vi "Swerve Drive 6181.vi"(0 "X":dbl(slide) scale=-1.0..1.0, 1 "Y":dbl(slide) scale=1.0..-1.0, 2 "Z":dbl(knob) scale=1.0..-1.0, 3 "Robot-Centric":bool, 4 "Auto Controls":bool) -> (5 "Avg Sensor Pos":dbl)   [LabVIEW 2019]
panel:
  in  "Robot Length":dbl=21.5
  in  "Robot Width":dbl=29.5
  # "SWERVE DRIVE\nVersion 3.1\n\nCory Lynch\nApple Pi Robotics\nTeam 2067"
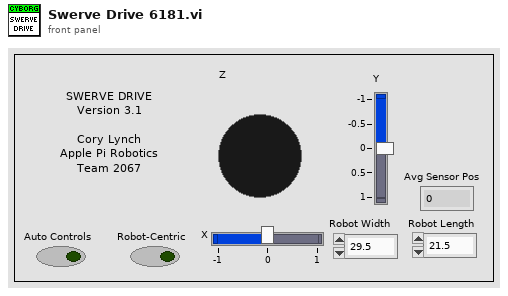
[diagram p1: front panel]
types:
  T1 = enum16{"Back Left", "Back Right", "Front Left", "Front Right"}
  T2 = cluster{"Yaw":dbl, "Roll":dbl, "Pitch":dbl, "Heading":dbl, "Fused Heading":dbl}
  T3 = typedef "WPI_MotorControlDeviceRef.ctl" = cluster{"DeviceStatus":errorcluster, "Type":T4, "PWM":cluster{"PWM Channel":T5, "DeadBand":T6}, "CAN":cluster{"Device Number":u8, "SetOutput VI Ref":variant, "GetOutput VI Ref":variant, "Enable VI Ref":variant, "Disable VI Ref":variant, "Data":variant}, "Invert":bool, "DIO PWM":cluster{"PWM \"Enable\" Channel":T5, "DIOChannel":T7, "PWM Rate":dbl}}
  T4 = typedef "WPI_MotorControlType.ctl" = enum16{"PWM", "CAN", "DIO PWM"}
  T5 = typedef "FPGA_DIOPWMChannel.ctl" = enum8{"PWM 0", "PWM 1", "PWM 2", "PWM 3", "PWM 4", "PWM 5", "PWM 6", "PWM 7", "PWM 8", "PWM 9", "PWM MXP 0", "PWM MXP 1", "PWM MXP 2", "PWM MXP 3", "PWM MXP 4", "PWM MXP 5", "PWM MXP 6", "PWM MXP 7", "PWM MXP 8", "PWM MXP 9", "Invalid"}
  T6 = typedef "WPI_PWMDeadband.ctl" = cluster{"Name":string, "maxPositivePwm":i32, "minPositivePwm":i32, "centerPwm":i32, "maxNegativePwm":i32, "minNegativePwm":i32, "angularRange":u16}
  T7 = typedef "FPGA_DIOChannel.ctl" = enum8{"DIO 0", "DIO 1", "DIO 2", "DIO 3", "DIO 4", "DIO 5", "DIO 6", "DIO 7", "DIO 8", "DIO 9", "DIO MXP 0", "DIO MXP 1", "DIO MXP 2", "DIO MXP 3", "DIO MXP 4", "DIO MXP 5", "DIO MXP 6", "DIO MXP 7", "DIO MXP 8", "DIO MXP 9", "DIO MXP 10", "DIO MXP 11", "DIO MXP 12", "DIO MXP 13", "DIO MXP 14", "DIO MXP 15", "SPI Port CS1", "SPI Port CS2", "SPI Port CS3", "SPI Port MISO", "SPI Port MOSI", "Invalid"}
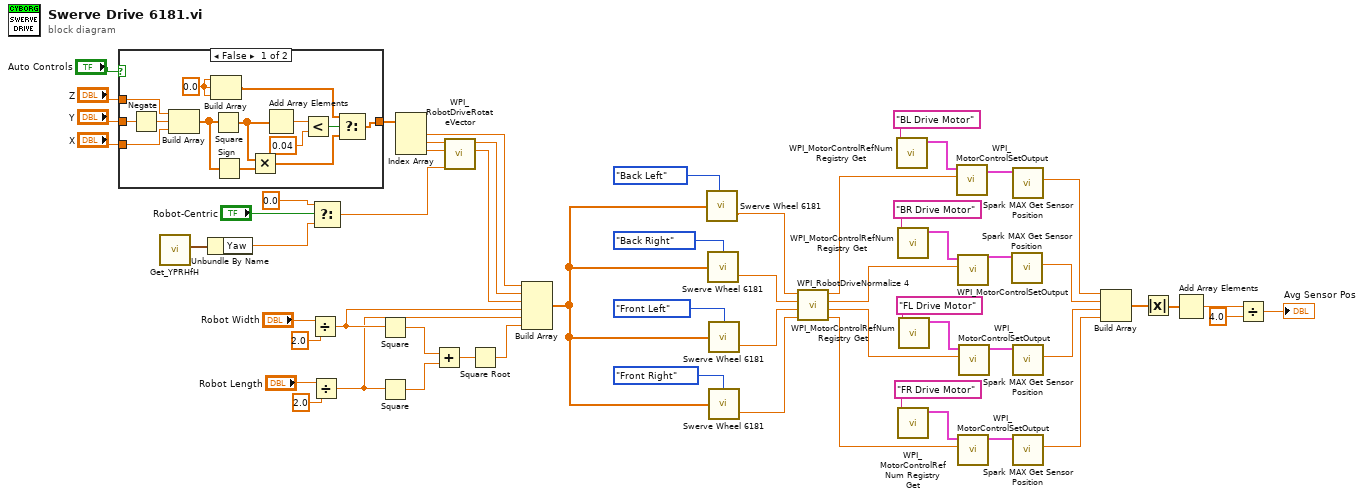
[diagram p0: block diagram]
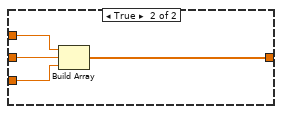
[diagram p2: hidden frame]
diagram:
  n1 = case shown="False" "Auto Controls" {
    tunnel: "Y" -> [w70 w76]
    tunnel: "X" -> [w64 w77]
    tunnel: "Z" -> [w60 w74]
    tunnel: [w61 w75] -> w35
    frame False {
      w68 = 0.0 ("element")
      n2 = Negate(x=w70) -> (-x=w63:dbl)
      n3 = Build Array(w60, w63, w64) -> (w67:dbl[])
      n4 = Build Array(w68, w68, w68) -> (w69:dbl[])
      n5 = Square(x=w67) -> (x^2=w65:dbl[])
      n6 = Sign(1:w67) -> (0:w66:dbl[])
      n7 = Multiply(x=w65, y=w66) -> (x*y=w62:dbl[])
      n8 = Add Array Elements(numeric array=w65) -> (sum=w73:dbl)
      n9 = Less?(x=w73, y=0.04 ("x")) -> (x < y?=w71:bool)
      n10 = Select(t=w69, s=w71, f=w62) -> (s? t:f=w61:dbl[])
    }
    frame True {
      n11 = Build Array(w74, w76, w77) -> (w75:dbl[])
    }
  }
  n12 = call <vilib>:"Get_YPRHfH.vi"() -> ("YRPHfH"=w26:T2)  [unwired: 11 in]
  n13 = Unbundle By Name(w26) -> ("Yaw"=w27:dbl)
  n14 = Divide(x="Robot Width", y=2.0) -> (x/y=w25:dbl)
  n15 = Divide(x="Robot Length", y=2.0) -> (x/y=w24:dbl)
  n16 = Select(t=0.0, s="Robot-Centric", f=w27) -> (s? t:f=w32:dbl)
  n17 = Square(x=w25) -> (x^2=w45:dbl)
  n18 = Square(x=w24) -> (x^2=w46:dbl)
  n19 = Index Array(array=w35) -> (element #1=w31:dbl, element #2=w36:dbl, element #3=w39:dbl)  [unwired: 3 in]
  n20 = Add(x=w45, y=w46) -> (x+y=w44:dbl)
  n21 = call <vilib>:"WPI_RobotDriveRotateVector.vi"("Angle"=w32, "X"=w39, "Y"=w36) -> ("X'"=w34:dbl, "Y'"=w30:dbl)  [unwired: 7 out]
  n22 = Square Root(x=w44) -> (sqrt(x)=w23:dbl)
  n23 = Build Array(w31, w30, w34, w25, w24, w23) -> (w15:dbl[])
  n24 = call "Swerve Wheel 6181.vi"("Wheel"=T1."Back Left", "Inputs"=w15) -> ("Speed"=w22:dbl)  [unwired: 3 in]
  n25 = call "Swerve Wheel 6181.vi"("Wheel"=T1."Back Right", "Inputs"=w15) -> ("Speed"=w20:dbl)  [unwired: 3 in]
  n26 = call "Swerve Wheel 6181.vi"("Wheel"=T1."Front Left", "Inputs"=w15) -> ("Speed"=w18:dbl)  [unwired: 3 in]
  n27 = call "Swerve Wheel 6181.vi"("Wheel"=T1."Front Right", "Inputs"=w15) -> ("Speed"=w16:dbl)  [unwired: 3 in]
  n28 = call <vilib>:"WPI_RobotDriveNormalize 4.vi"("D"=w16, "C"=w18, "B"=w20, "A"=w22) -> ("D'"=w48:dbl, "C'"=w49:dbl, "B'"=w50:dbl, "A'"=w51:dbl)
  n29 = call <vilib>:"WPI_MotorControlRefNum Registry Get.vi"("refnum name"="BL Drive Motor") -> ("MotorControlDevRef"=w59:T3)  [unwired: 9 in, 1 out]
  n30 = call <vilib>:"WPI_MotorControlRefNum Registry Get.vi"("refnum name"="BR Drive Motor") -> ("MotorControlDevRef"=w56:T3)  [unwired: 9 in, 1 out]
  n31 = call <vilib>:"WPI_MotorControlRefNum Registry Get.vi"("refnum name"="FR Drive Motor") -> ("MotorControlDevRef"=w52:T3)  [unwired: 9 in, 1 out]
  n32 = call <vilib>:"WPI_MotorControlRefNum Registry Get.vi"("refnum name"="FL Drive Motor") -> ("MotorControlDevRef"=w55:T3)  [unwired: 9 in, 1 out]
  n33 = call <vilib>:"WPI_MotorControlSetOutput.vi"("Output"=w51, "MotorControlDevRef"=w59) -> ("MotorControlDevRef"=w13:T3)  [unwired: 7 in, 2 out]
  n34 = call <vilib>:"WPI_MotorControlSetOutput.vi"("Output"=w50, "MotorControlDevRef"=w56) -> ("MotorControlDevRef"=w12:T3)  [unwired: 7 in, 2 out]
  n35 = call <vilib>:"WPI_MotorControlSetOutput.vi"("Output"=w48, "MotorControlDevRef"=w52) -> ("MotorControlDevRef"=w10:T3)  [unwired: 7 in, 2 out]
  n36 = call <vilib>:"WPI_MotorControlSetOutput.vi"("Output"=w49, "MotorControlDevRef"=w55) -> ("MotorControlDevRef"=w11:T3)  [unwired: 7 in, 2 out]
  n37 = call <vilib>:"Spark MAX Get Sensor Position.vi"("MotorControlDevRef in"=w12) -> ("Sensor Position"=w7:dbl)  [unwired: 7 in, 3 out]
  n38 = call <vilib>:"Spark MAX Get Sensor Position.vi"("MotorControlDevRef in"=w13) -> ("Sensor Position"=w6:dbl)  [unwired: 7 in, 3 out]
  n39 = call <vilib>:"Spark MAX Get Sensor Position.vi"("MotorControlDevRef in"=w11) -> ("Sensor Position"=w8:dbl)  [unwired: 7 in, 3 out]
  n40 = call <vilib>:"Spark MAX Get Sensor Position.vi"("MotorControlDevRef in"=w10) -> ("Sensor Position"=w9:dbl)  [unwired: 7 in, 3 out]
  n41 = Build Array(w6, w7, w8, w9) -> (w5:dbl[])
  n42 = Absolute Value(x=w5) -> (abs(x)=w4:dbl[])
  n43 = Add Array Elements(numeric array=w4) -> (sum=w3:dbl)
  n44 = Divide(x=w3, y=4.0) -> (x/y=→"Avg Sensor Pos":dbl)
